vi "CreateScanList.vi"(7 "Slot":T1, 11 "Channels":bool[](array[boolean])) -> (3 "Channel List":string)   [LabVIEW 2012, in "Keithley-7001.lvlib"]
uses:
  Public/Controls/Slot.ctl
  Keithley-7001.lvlib
panel:
  # "33"
  # "34"
  # "35"
  # "1"
  # "2"
  # "3"
  # "4"
  # "5"
  # "6"
  # "7"
  # "8"
  # "9"
  # "10"
  # "11"
  # "12"
  # "13"
  # "14"
  # "15"
  # "16"
  # "17"
  # "18"
  # "19"
  # "20"
  # "21"
  # "22"
  # "23"
  # "24"
  # "25"
  # "26"
  # "27"
  # "28"
  # "29"
  # "30"
  # "31"
  # "32"
  # "36"
  # "37"
  # "38"
  # "39"
  # "40"
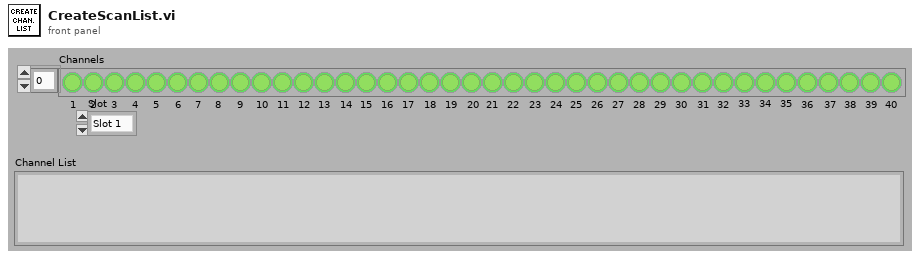
[diagram p1: front panel]
types:
  T1 = typedef "Keithley-7001.lvlib/Slot.ctl" = enum16{"Slot 1", "Slot 2"}
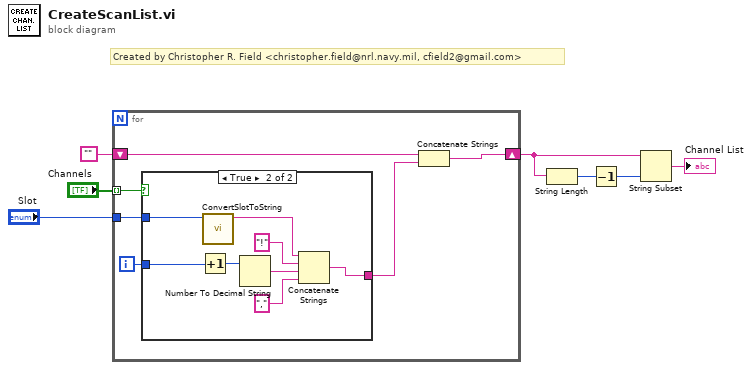
[diagram p0: block diagram]
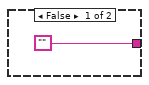
[diagram p2: hidden frame]
diagram:
  # "Created by Christopher R. Field <christopher.field@nrl.navy.mil, cfield2@gmail.com>"
  n1 = for {
    tunnel: "Channels" -> [w11] mode=indexing
    shift-right: [w9] -> w5
    shift-left: "" -> [w12]
    tunnel: "Slot" -> [w8]
    i -> [w13]
    n2 = case shown="True" w11 {
      tunnel: w13 -> [_ w22]
      tunnel: ["" w18] -> w10
      tunnel: w8 -> [_ w15]
      frame False {
      }
      frame True {
        n3 = Increment(x=w22) -> (x+1=w21:i32)
        n4 = call "ConvertSlotToString.vi"("Slot"=w15) -> ("Slot"=w16:string)  [unwired: 10 in]
        n5 = Number To Decimal String(number=w21) -> (decimal integer string=w20:string)  [unwired: 1 in]
        n6 = Concatenate Strings(w16, "!", w20, ",") -> (w18:string)
      }
    }
    n7 = Concatenate Strings(w12, w10) -> (w9:string)
  }
  n8 = String Length(string=w5) -> (length=w4:i32)
  n9 = Decrement(x=w4) -> (x-1=w3:i32)
  n10 = String Subset(string=w5, length (rest)=w3) -> (substring=→"Channel List":string)  [unwired: 1 in]
